vi "AB_Engine_Reassign_Destinations_For_Preserve_Hierarchy.vi"(4 "newPath":path, 5 "PPL Table":variant, 6 "parentIndex in":i32, 7 "source index":i32, 8 "error in (no error)":errorcluster, 9 "source":refnum<class "AB_Source.lvclass">, 10 "destinations in":refnum<class "AB_Destination.lvclass">[](array[class]), 11 "sources in":refnum<class "AB_Source.lvclass">[](array[class])) -> (0 "error out":errorcluster, 2 "destination out":refnum<class "AB_Destination.lvclass">[](array[class]), 3 "sources out":refnum<class "AB_Source.lvclass">[](array[class]))   [LabVIEW 2020]
uses:
  <vilib>/AppBuilder/AB_Classes/Destination/AB_Destination.lvclass
  <vilib>/AppBuilder/AB_Classes/Source/AB_Source.lvclass
  <vilib>/AppBuilder/Engine/AB_Engine_PPL_Source_Index.ctl
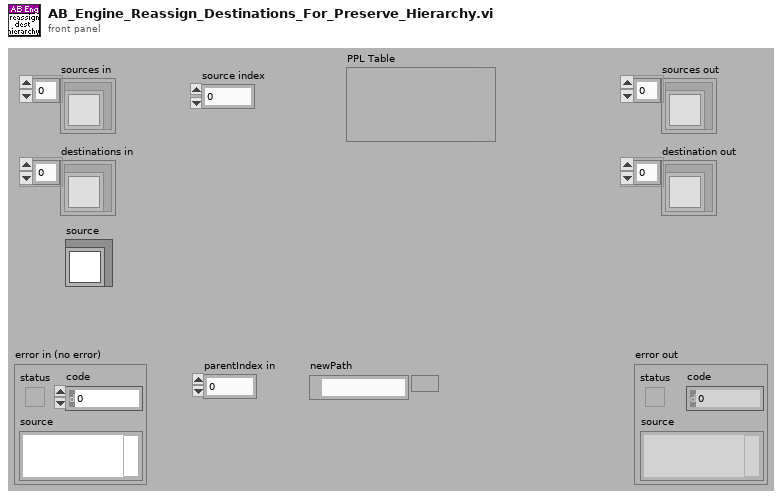
[diagram p1: front panel]
types:
  T1 = typedef "AB_Source.ctl" = cluster{"path":path, "itemID":string, "parentIndex":i32, "sourceInclusion":T2, "destinationIndex":i32, "properties":T3[], "newName":string, "lvfile":bool, "valid":bool, "eng_inBuild":bool, "eng_isNonVILink":bool, "Amalgamation":bool, "Amalgamation Piece":bool, "eng_delimitedName":string, "preventRename":bool}
  T2 = typedef "AB_Source_Inclusion.ctl" = enum16{"IncludeIfReferenced", "Include", "Exclude", "TopLevel"}
  T3 = typedef "AB_Source_Properties.ctl" = cluster{"sourcePropertyType":T4, "value":variant}
  T4 = typedef "AB_Source_Property_Type.ctl" = enum16{"Remove block diagram", "Remove front panel", "Password", "Window has title bar", "Show menu bar", "Show vertical scroll bar", "Show horizontal scroll bar", "Show toolbar", "Show Abort button", "Show fp when called", "Window behavior", "Allow user to close window", "Window run-time position", "Run when opened", "Allow debugging", "Auto error handling", "Generate guard code", "Use stack variables", "Expression folding", "Integer only", "Inline subVI"}
  T5 = typedef "AB_Engine_PPL_Source_Index.ctl" = cluster{"path":path, "source index":i32, "PPL?":bool}
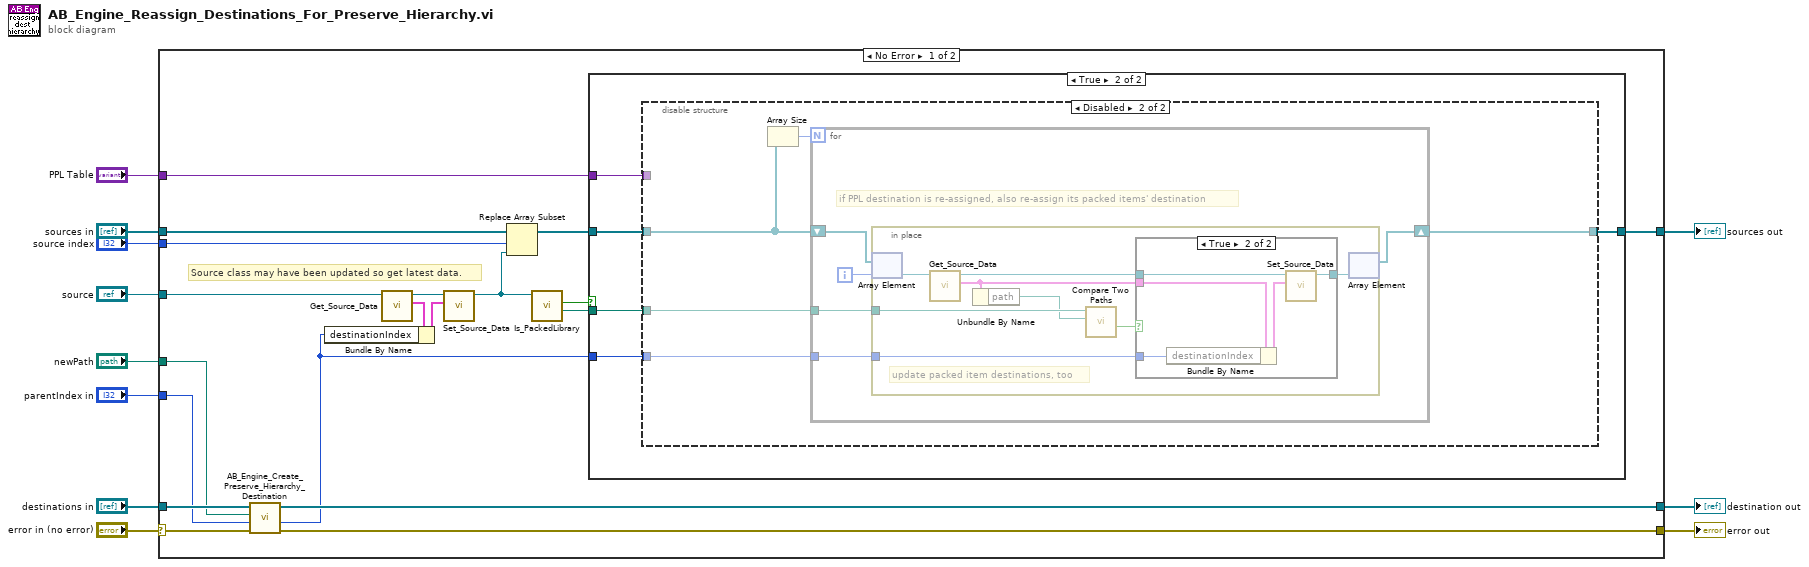
[diagram p0: block diagram]
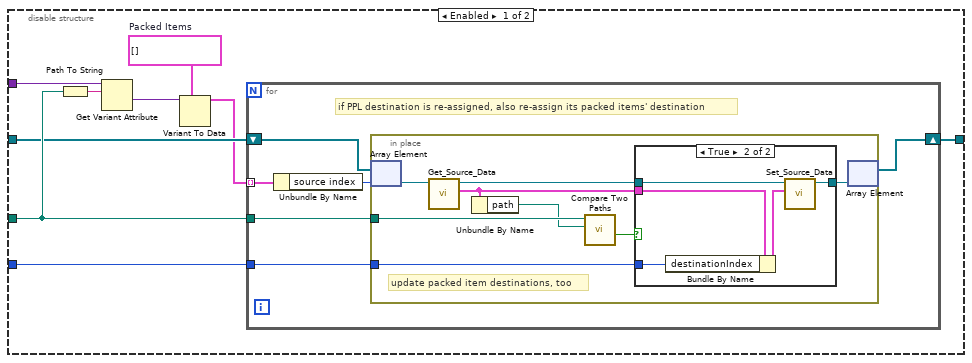
[diagram p3: hidden frame]
diagram:
  n1 = case shown="No Error" "error in (no error)" {
    selector: "error in (no error)" -> [w21 w92]
    tunnel: [w20 w92] -> w6
    tunnel: [w24 w91] -> w8
    tunnel: "destinations in" -> [w25 w91]
    tunnel: "newPath" -> [w23 _]
    tunnel: "parentIndex in" -> [w22 _]
    tunnel: "sources in" -> [w27 w90]
    tunnel: [w15 w90] -> w4
    tunnel: "source" -> [w26 _]
    tunnel: "source index" -> [w14 _]
    tunnel: "PPL Table" -> [w12 _]
    frame No Error {
      # "Source class may have been updated so get latest data."
      n2 = call <vilib>:"AB_Engine_Create_Preserve_Hierarchy_Destination.vi"("error in (no error)"=w21, "parentIndex in"=w22, "newPath"=w23, "destinations in"=w25) -> ("error out"=w20:errorcluster, "destinationIndex out"=w13:i32, "destination out"=w24:refnum<class "AB_Destination.lvclass">[])  [unwired: 5 out]
      n3 = call <vilib>:"Get_Source_Data.vi"("Class in"=w26) -> ("data"=w28:T1, "Class out"=w29:refnum<class "AB_Source.lvclass">)  [unwired: 1 in, 8 out]
      n4 = Bundle By Name(cluster=w28, "destinationIndex"=w13) -> (w30:T1)
      n5 = call <vilib>:"Set_Source_Data.vi"("data"=w30, "Class in"=w29) -> ("Class out"=w19:refnum<class "AB_Source.lvclass">)  [unwired: 1 in, 8 out]
      n6 = Replace Array Subset(array=w27, new element=w19, index=w14) -> (w16:refnum<class "AB_Source.lvclass">[])
      n7 = call <vilib>:"Is_PackedLibrary.vi"("AB_Source in"=w19) -> ("path"=w17:path, "PPL?"=w18:bool)  [unwired: 7 in, 2 out]
      n8 = case shown="True" w18 {
        tunnel: w17 -> [_ w35]
        tunnel: w16 -> [w31 w33]
        tunnel: [w31 w36] -> w15
        tunnel: w13 -> [_ w34]
        tunnel: w12 -> [_ w32]
        frame False {
        }
        frame True {
          n9 = disable-structure shown="Disabled" {
            disable-tunnel: [w45 w70] -> w36
            disable-tunnel: w35 -> [w44 w69]
            disable-tunnel: w34 -> [w43 w68]
            disable-tunnel: w33 -> [w42 w66]
            disable-tunnel: w32 -> [w41 _]
            frame Enabled {
              w38 = T5[] []  # Packed Items
              n10 = Path To String(path=w44) -> (string=w40:string)
              n11 = Get Variant Attribute(Variant=w41, name=w40) -> (value=w39:variant)  [unwired: 2 in, 3 out]
              n12 = Variant To Data(type=w38, Variant=w39) -> (data=w37:T5[])  [unwired: 1 in, 1 out]
              n13 = for {
                tunnel: w44 -> [w51]
                tunnel: w43 -> [w50]
                shift-right: [w48] -> w45
                shift-left: w42 -> [w49]
                tunnel: w37 -> [w47] mode=indexing
                # "if PPL destination is re-assigned, also re-assign its packed items' destination"
                n14 = Unbundle By Name(w47) -> ("source index"=w46:i32)
                n15 = in-place {
                  in-place-border: w51 -> [w57]
                  in-place-border: w50 -> [w52]
                  # "update packed item destinations, too"
                  n16 = in-place-array #1(w49, w46) -> (w58:refnum<class "AB_Source.lvclass">)
                  n17 = call <vilib>:"Get_Source_Data.vi"("Class in"=w58) -> ("data"=w54:T1, "Class out"=w59:refnum<class "AB_Source.lvclass">)  [unwired: 1 in, 8 out]
                  n18 = Unbundle By Name(w54) -> ("path"=w56:path)
                  n19 = call <vilib>:"Compare Two Paths.vi"("Path 2"=w56, "Path 1"=w57) -> ("Path 2 Relative to Path 1?"=w55:bool)  [unwired: 6 in, 3 out]
                  n20 = case shown="True" w55 {
                    tunnel: w59 -> [w60 w65]
                    tunnel: w54 -> [_ w63]
                    tunnel: [w60 w62] -> w53
                    tunnel: w52 -> [_ w61]
                    frame False {
                    }
                    frame True {
                      n21 = Bundle By Name(cluster=w63, "destinationIndex"=w61) -> (w64:T1)
                      n22 = call <vilib>:"Set_Source_Data.vi"("data"=w64, "Class in"=w65) -> ("Class out"=w62:refnum<class "AB_Source.lvclass">)  [unwired: 1 in, 8 out]
                    }
                  }
                  n23 = in-place-array #1(w53) -> (w48:refnum<class "AB_Source.lvclass">[])  [unwired: 1 out]
                }
              }
            }
            frame Disabled {
              n24 = Array Size(array=w66) -> (size(s)=w67:i32)
              n25 = for {
                N: w67 -> [_]
                tunnel: w69 -> [w75]
                tunnel: w68 -> [w74]
                shift-right: [w72] -> w70
                shift-left: w66 -> [w73]
                i -> [w71]
                # "if PPL destination is re-assigned, also re-assign its packed items' destination"
                n26 = in-place {
                  in-place-border: w75 -> [w81]
                  in-place-border: w74 -> [w76]
                  # "update packed item destinations, too"
                  n27 = in-place-array #2(w73, w71) -> (w82:refnum<class "AB_Source.lvclass">)
                  n28 = call <vilib>:"Get_Source_Data.vi"("Class in"=w82) -> ("data"=w78:T1, "Class out"=w83:refnum<class "AB_Source.lvclass">)  [unwired: 1 in, 8 out]
                  n29 = Unbundle By Name(w78) -> ("path"=w80:path)
                  n30 = call <vilib>:"Compare Two Paths.vi"("Path 2"=w80, "Path 1"=w81) -> ("Path 2 Relative to Path 1?"=w79:bool)  [unwired: 6 in, 3 out]
                  n31 = case shown="True" w79 {
                    tunnel: w83 -> [w84 w89]
                    tunnel: w78 -> [_ w87]
                    tunnel: [w84 w86] -> w77
                    tunnel: w76 -> [_ w85]
                    frame False {
                    }
                    frame True {
                      n32 = Bundle By Name(cluster=w87, "destinationIndex"=w85) -> (w88:T1)
                      n33 = call <vilib>:"Set_Source_Data.vi"("data"=w88, "Class in"=w89) -> ("Class out"=w86:refnum<class "AB_Source.lvclass">)  [unwired: 1 in, 8 out]
                    }
                  }
                  n34 = in-place-array #2(w77) -> (w72:refnum<class "AB_Source.lvclass">[])  [unwired: 1 out]
                }
              }
            }
          }
        }
      }
    }
    frame Error {
    }
  }
  "error out" <- w6
  "destination out" <- w8
  "sources out" <- w4
